vi "Transmission.vi"() -> ()   [LabVIEW 2016, in "Beamline Sections - Common.lvlib"]
uses:
  Beamline Sections - Common.lvlib
  <vilib>/Instr/_visa.llb/VISA Open Access Mode.ctl
  main/save load/saveload.ctl
panel:
  out "error out 3":errorcluster
  out "error out":errorcluster
  out "error out 2":errorcluster
  out "appended array":bool[](array[boolean])
  in  "Tab Control":enum32{"Control", "Readbacks"}(tab)
  in  "ExB Electric":dbl(knob) min=0.0 max=200.0 scale=33.0..36.0
  out "Trans Steerer Y Read":dbl format="%#.3g"
  out "Trans Steerer X Read":dbl format="%#.3g"
  in  "Transmission Y steerer":dbl(knob) min=-10.0 max=10.0 scale=-10.0..10.0
  in  "Transmission Quad A":dbl(knob) min=0.0 max=200.0 scale=5.0..120.0
  out "Switch magnet Range":bool=TRUE
  out "Switch magnet readback":dbl(graph)=0.8365
  in  "Switch magnet power supply":dbl(slide)=0.8365 min=0.0 max=1.6 scale=0.4..0.7
  in  "Transmission X steerer":dbl(knob) min=-10.0 max=10.0 scale=-10.0..10.0
  out "Transmission\n Steerer range":bool
  out "He Trans mission quad Range":bool
  in  "Transmission Quad B":dbl(knob) min=0.0 max=200.0 scale=6.0..120.0
  in  "stop":bool
  out "ExB":bool
  out "ExB Voltage Read-":dbl format="%#.3g"
  in  "ExB Magnet":dbl
  in  "Cluster":T1
  out "Switch magnet cup":bool
  out "ExB Voltage Read +":dbl format="%#.3g"
  out "read current quad a":string
  out "read voltage quad A":string
  out "read voltage Quad B":string
  out "read current quad B":string
  out "ExB +READ I":dbl
  out "ExB - I":dbl
  out "Trans steer +X I":dbl
  out "Trans steer -X  I":dbl
  out "Trans steer +Y I":dbl
  out "Trans steer -Y I":dbl
  out "Trans steer +X":dbl
  out "Trans steer -X":dbl
  out "Trans steer +Y":dbl
  out "Trans steer -Y":dbl
  out "Trans steer +X Set":dbl
  out "Trans steer -X Set":dbl
  out "Trans steer +Y Set":dbl
  out "Trans steer -Y Set":dbl
  out "Switch magnet field readback":dbl=0.8365 min=0.0 max=1.6
  out "analyze power supply":dbl
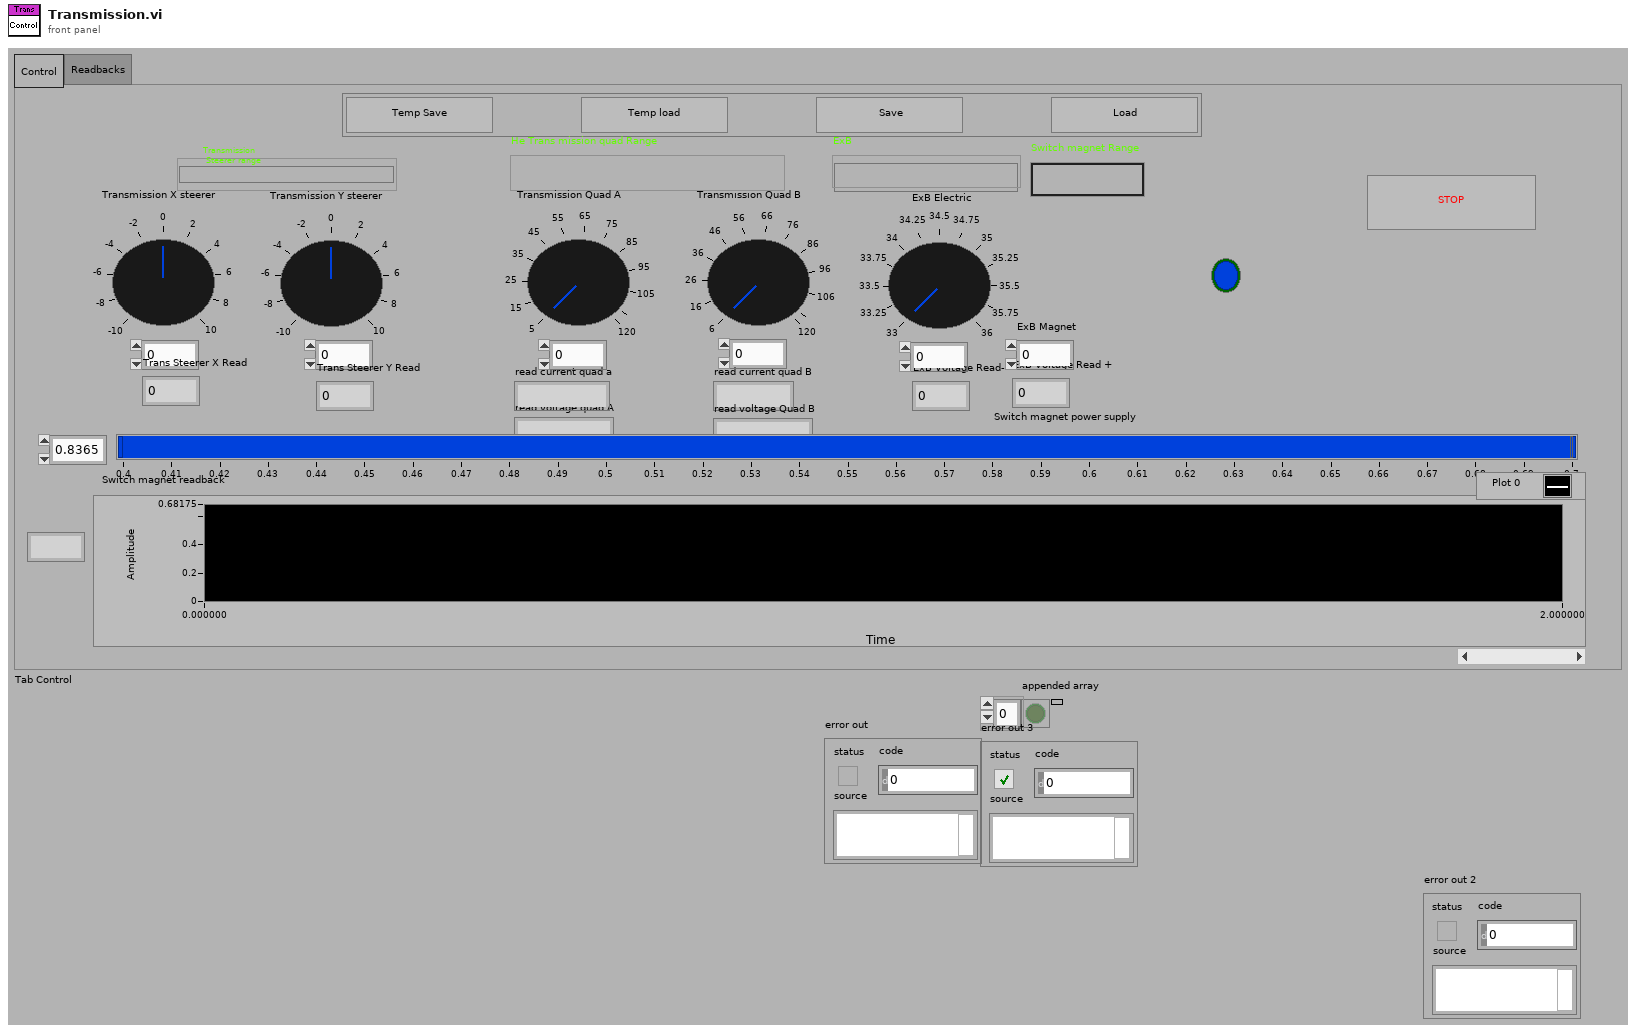
[diagram p1: front panel]
types:
  T1 = typedef "main.lvlib/saveload.ctl" = cluster{"OK Button":bool, "OK Button 2":bool, "OK Button 3":bool, "OK Button 4":bool}
  T2 = typedef "VISA Open Access Mode.ctl" = u32
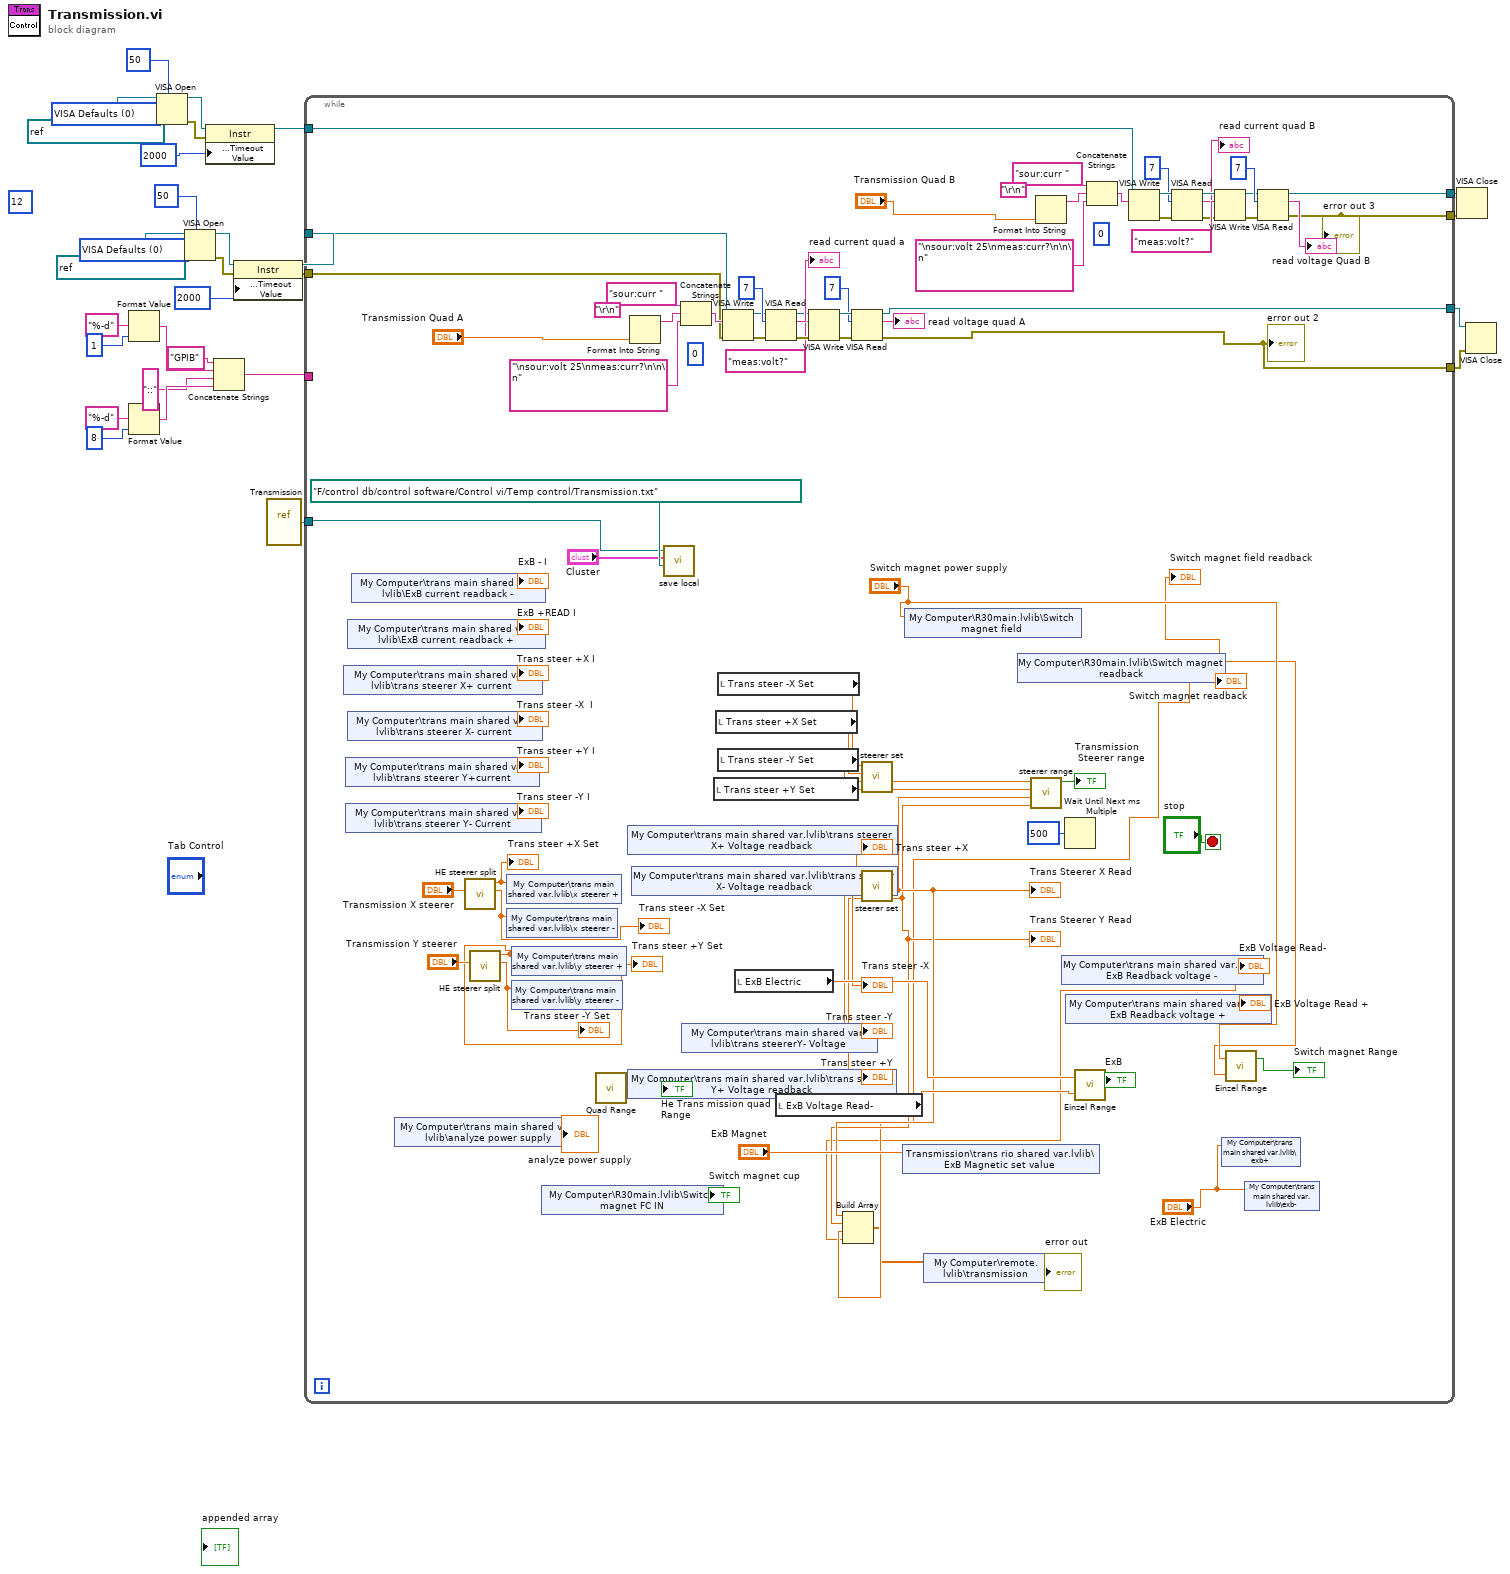
[diagram p0: block diagram]
diagram:
  w7 = T2 0 items=["VISA Defaults"=0, "Exclusive Lock"=1, "Load Configured Settings"=4] ("Access Mode")
  w19 = T2 0 items=["VISA Defaults"=0, "Exclusive Lock"=1, "Load Configured Settings"=4] ("Access Mode")
  (unwired) u16 12 ("Device\nAddress(1)")
  n1 = Format Value(format string="%-d", value (0)=u16 1 ("Controller\nAddress(0) 2")) -> (output string=w27:string)  [unwired: 1 in]
  n2 = Format Value(format string="%-d", value (0)=u16 8 ("Device\nAddress(1) 2")) -> (output string=w22:string)  [unwired: 1 in]
  n3 = VISA Open(timeout (0)=u32 50 ("VISA Open timeout (0)"), access mode=w7, VISA resource name=refnum<visa-resource-name> "GPIB2::12::INSTR" ("VISA GPIB Resource")) -> (VISA resource name=w10:refnum<visa-resource-name>, error out=w11:errorcluster)  [unwired: 2 in]
  n4 = VISA Open(timeout (0)=u32 50 ("VISA Open timeout (0)"), access mode=w19, VISA resource name=refnum<visa-resource-name> "GPIB2::8::INSTR" ("VISA GPIB Resource")) -> (VISA resource name=w15:refnum<visa-resource-name>, error out=w14:errorcluster)  [unwired: 2 in]
  n5 = property class="Instr"(reference=w10, error in=w11, "General Settings:Timeout Value"=u32 2000) -> (reference out=w5:refnum<visa-resource-name>)  [unwired: 1 out]
  n6 = Concatenate Strings("GPIB", w27, "::", w22) -> (w20:string)
  n7 = property class="Instr"(reference=w15, error in=w14, "General Settings:Timeout Value"=u32 2000) -> (reference out=w12:refnum<visa-resource-name>, error out=w13:errorcluster)
  n8 = vi-ref "Transmission.vi"() -> (w29:refnum<vi>)
  n9 = while {
    tunnel: w29 -> [w101]
    tunnel: w20 -> [_]
    tunnel: w12 -> [w71]
    tunnel: w13 -> [w62]
    tunnel: w5 -> [w46]
    tunnel: [w43] -> w4
    tunnel: [w42] -> w3
    tunnel: [w41] -> w2
    tunnel: [w40] -> w1
    stop <- "stop" stop-if-true
    (unwired) "\r\n"
    (unwired) i16 0 ("mode (0)")
    (unwired) "\r\n"
    (unwired) i16 0 ("mode (0)")
    n10 = shared-variable "My Computer\\trans main shared var.lvlib\\trans steerer X+ current"() -> (→"Trans steer +X I":dbl)  [unwired: 1 in, 1 out]
    n11 = shared-variable "My Computer\\trans main shared var.lvlib\\trans steerer Y+current"() -> (→"Trans steer +Y I":dbl)  [unwired: 1 in, 1 out]
    n12 = shared-variable "My Computer\\trans main shared var.lvlib\\trans steerer Y- Current"() -> (→"Trans steer -Y I":dbl)  [unwired: 1 in, 1 out]
    n13 = shared-variable "My Computer\\trans main shared var.lvlib\\ExB current readback +"() -> (→"ExB +READ I":dbl)  [unwired: 1 in, 1 out]
    n14 = shared-variable "My Computer\\trans main shared var.lvlib\\trans steerer X- current"() -> (→"Trans steer -X  I":dbl)  [unwired: 1 in, 1 out]
    n15 = shared-variable "My Computer\\trans main shared var.lvlib\\ExB current readback -"() -> (→"ExB - I":dbl)  [unwired: 1 in, 1 out]
    n16 = shared-variable "My Computer\\trans main shared var.lvlib\\analyze power supply"() -> (→"analyze power supply":dbl)  [unwired: 1 in, 1 out]
    n17 = call "HE steerer split.vi"("Steerer in"="Transmission X steerer") -> ("Steerer +"=w37:dbl, "Steerer -"=w82:dbl)  [unwired: 7 in]
    "Trans steer +X Set" <- w37
    "Trans steer -X Set" <- w82
    n18 = call "HE steerer split.vi"("Steerer in"="Transmission Y steerer") -> ("Steerer +"=w80:dbl, "Steerer -"=w81:dbl)  [unwired: 7 in]
    "Trans steer +Y Set" <- w80
    "Trans steer -Y Set" <- w81
    n19 = shared-variable "My Computer\\trans main shared var.lvlib\\x steerer +"(w37) -> ()  [unwired: 1 in, 1 out]
    n20 = shared-variable "My Computer\\trans main shared var.lvlib\\x steerer -"(w82) -> ()  [unwired: 1 in, 1 out]
    n21 = shared-variable "My Computer\\trans main shared var.lvlib\\y steerer +"(w80) -> ()  [unwired: 1 in, 1 out]
    n22 = shared-variable "My Computer\\trans main shared var.lvlib\\y steerer -"(w81) -> ()  [unwired: 1 in, 1 out]
    n23 = shared-variable "My Computer\\R30main.lvlib\\Switch magnet FC IN"() -> (→"Switch magnet cup":bool)  [unwired: 1 in, 1 out]
    n24 = call "Quad Range.vi"() -> ("Quad range?"=→"He Trans mission quad Range":bool)  [unwired: 4 in]
    n25 = shared-variable "My Computer\\trans main shared var.lvlib\\trans steerer X+ Voltage readback"() -> (w95:dbl)  [unwired: 1 in, 1 out]
    "Trans steer +X" <- w95
    n26 = shared-variable "My Computer\\trans main shared var.lvlib\\trans steerer Y+ Voltage readback"() -> (w93:dbl)  [unwired: 1 in, 1 out]
    "Trans steer +Y" <- w93
    n27 = Format Into String("Transmission Quad A") -> (resulting string=w77:string)  [unwired: 3 in, 1 out]
    n28 = shared-variable "My Computer\\trans main shared var.lvlib\\trans steerer X- Voltage readback"() -> (w94:dbl)  [unwired: 1 in, 1 out]
    "Trans steer -X" <- w94
    n29 = call "save local.vi"("file path (use dialog)"=path "F:/control db/control software/Control vi/Temp control/Transmission.txt", "Ring"="Cluster", "VI Refnum"=w101) -> ()  [unwired: 2 out]
    n30 = Concatenate Strings("sour:curr " ("string"), w77, "\nsour:volt 25\nmeas:curr?\n\n\n" ("write buffer")) -> (w72:string)
    n31 = shared-variable "My Computer\\trans main shared var.lvlib\\trans steererY- Voltage"() -> (w92:dbl)  [unwired: 1 in, 1 out]
    "Trans steer -Y" <- w92
    n32 = local read "Trans steer +Y Set"() -> (w110:dbl)
    n33 = local read "Trans steer +X Set"() -> (w108:dbl)
    n34 = local read "Trans steer -X Set"() -> (w107:dbl)
    n35 = local read "Trans steer -Y Set"() -> (w109:dbl)
    n36 = VISA Write(VISA resource name=w71, write buffer=w72, error in (no error)=w62) -> (VISA resource name out=w73:refnum<visa-resource-name>, error out=w74:errorcluster)  [unwired: 1 out]
    n37 = local read "ExB Electric"() -> (w104:dbl)
    n38 = VISA Read(VISA resource name=w73, byte count=u32 7, error in (no error)=w74) -> (VISA resource name out=w67:refnum<visa-resource-name>, read buffer=→"read current quad a":string, error out=w66:errorcluster)  [unwired: 1 out]
    n39 = local read "ExB Voltage Read-"() -> (w105:dbl)
    n40 = VISA Write(VISA resource name=w67, write buffer="meas:volt?", error in (no error)=w66) -> (VISA resource name out=w69:refnum<visa-resource-name>, error out=w64:errorcluster)  [unwired: 1 out]
    n41 = VISA Read(VISA resource name=w69, byte count=u32 7, error in (no error)=w64) -> (VISA resource name out=w40:refnum<visa-resource-name>, read buffer=→"read voltage quad A":string, error out=w41:errorcluster)  [unwired: 1 out]
    "error out 2" <- w41
    n42 = call "steerer set.vi"("Injector image X  -"=w107, "Injector image X +"=w108, "Injector image Y  -"=w109, "Injector image Y +"=w110) -> ("Steerer X"=w100:dbl, "Steerer Y"=w99:dbl)  [unwired: 4 out]
    n43 = call "steerer set.vi"("Injector image X  -"=w94, "Injector image X +"=w95, "Injector image Y  -"=w92, "Injector image Y +"=w93) -> ("Steerer X"=w36:dbl, "Steerer Y"=w35:dbl)  [unwired: 4 out]
    "Trans Steerer X Read" <- w36
    "Trans Steerer Y Read" <- w35
    n44 = shared-variable "Transmission\\trans rio shared var.lvlib\\ExB Magnetic set value"("ExB Magnet") -> ()  [unwired: 1 in, 1 out]
    n45 = shared-variable "My Computer\\R30main.lvlib\\Switch magnet field"("Switch magnet power supply") -> ()  [unwired: 1 in, 1 out]
    n46 = shared-variable "My Computer\\R30main.lvlib\\Switch magnet readback"() -> (w34:dbl)  [unwired: 1 in, 1 out]
    "Switch magnet readback" <- w34
    "Switch magnet field readback" <- w34
    n47 = call "steerer range.vi"("Steerer Y Voltage"=w35, "Steerer X Voltage"=w36, "Steerer Set Y"=w99, "Steerer X Set"=w100) -> ("Steerer within range"=→"Transmission\n Steerer range":bool)  [unwired: 3 out]
    n48 = Format Into String("Transmission Quad B") -> (resulting string=w49:string)  [unwired: 3 in, 1 out]
    n49 = shared-variable "My Computer\\trans main shared var.lvlib\\ExB Readback voltage -"() -> (w33:dbl)  [unwired: 1 in, 1 out]
    "ExB Voltage Read-" <- w33
    n50 = Build Array(w36, w35, w34, w33) -> (w32:dbl[])
    n51 = shared-variable "My Computer\\remote.lvlib\\transmission"(w32) -> (error out=→"error out":errorcluster)  [unwired: 1 in]
    n52 = Wait Until Next ms Multiple(millisecond multiple=u32 500) -> ()  [unwired: 1 out]
    n53 = shared-variable "My Computer\\trans main shared var.lvlib\\ExB Readback voltage +"() -> (→"ExB Voltage Read +":dbl)  [unwired: 1 in, 1 out]
    n54 = call "Einzel Range.vi"("Inj image Readback"=w105, "Inj image Einzel Set"=w104) -> ("Einzel  Range"=→"ExB":bool)  [unwired: 1 out]
    n55 = Concatenate Strings("sour:curr " ("string"), w49, "\nsour:volt 25\nmeas:curr?\n\n\n" ("write buffer")) -> (w53:string)
    n56 = VISA Write(VISA resource name=w46, write buffer=w53) -> (VISA resource name out=w52:refnum<visa-resource-name>, error out=w51:errorcluster)  [unwired: 1 in, 1 out]
    n57 = VISA Read(VISA resource name=w52, byte count=u32 7, error in (no error)=w51) -> (VISA resource name out=w56:refnum<visa-resource-name>, read buffer=→"read current quad B":string, error out=w57:errorcluster)  [unwired: 1 out]
    n58 = VISA Write(VISA resource name=w56, write buffer="meas:volt?", error in (no error)=w57) -> (VISA resource name out=w54:refnum<visa-resource-name>, error out=w59:errorcluster)  [unwired: 1 out]
    n59 = shared-variable "My Computer\\trans main shared var.lvlib\\exb+"("ExB Electric") -> ()  [unwired: 1 in, 1 out]
    n60 = call "Einzel Range.vi"("Inj image Readback"=w34, "Inj image Einzel Set"="Switch magnet power supply") -> ("Einzel  Range"=→"Switch magnet Range":bool)  [unwired: 1 out]
    n61 = shared-variable "My Computer\\trans main shared var.lvlib\\exb-"("ExB Electric") -> ()  [unwired: 1 in, 1 out]
    n62 = VISA Read(VISA resource name=w54, byte count=u32 7, error in (no error)=w59) -> (VISA resource name out=w43:refnum<visa-resource-name>, read buffer=→"read voltage Quad B":string, error out=w42:errorcluster)  [unwired: 1 out]
    "error out 3" <- w42
  }
  n63 = VISA Close(VISA resource name=w4, error in (no error)=w3) -> ()  [unwired: 1 out]
  n64 = VISA Close(VISA resource name=w1, error in (no error)=w2) -> ()  [unwired: 1 out]
